vi "Find_Row_Shaft-mm.vi"(0 "Basic Size":dbl, 5 "error in":errorcluster) -> (6 "Row":i32, 8 "error out":errorcluster)   [LabVIEW 2023]
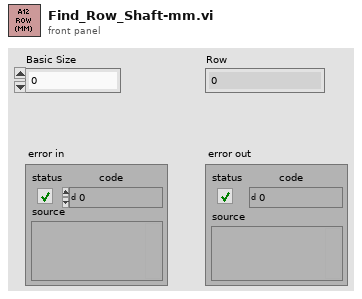
[diagram p1: front panel]
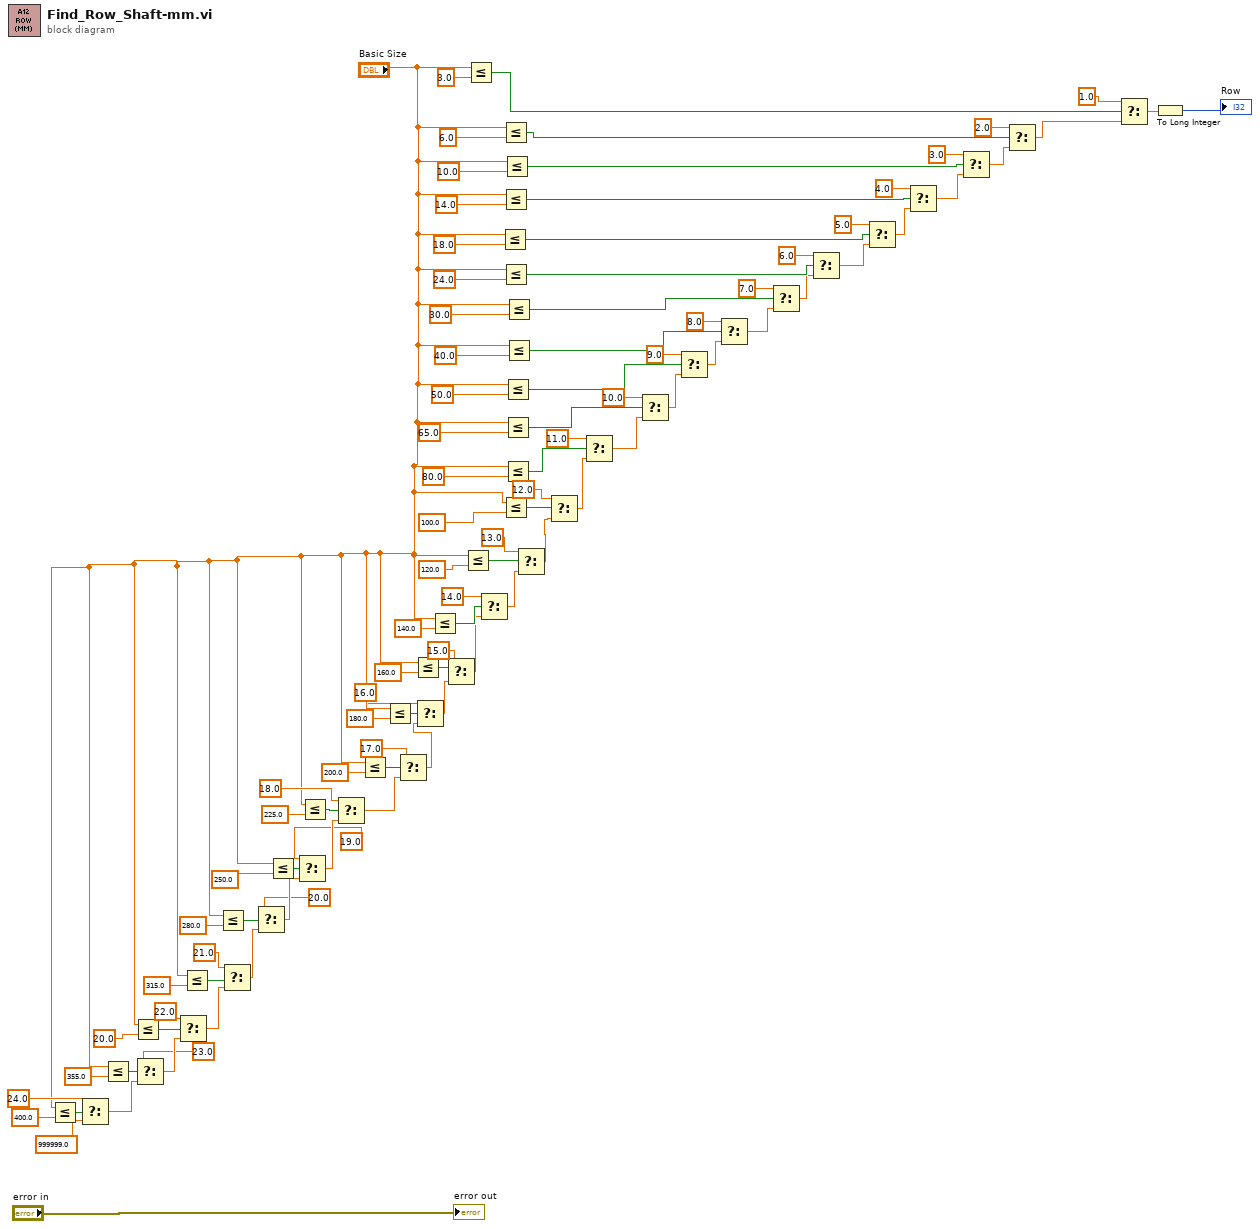
[diagram p0: block diagram]
diagram:
  n1 = Less Or Equal?(x="Basic Size", y=400.0) -> (x <= y?=w8:bool)
  n2 = Select(t=24.0, s=w8, f=999999.0) -> (s? t:f=w10:dbl)
  n3 = Less Or Equal?(x="Basic Size", y=355.0) -> (x <= y?=w13:bool)
  n4 = Less Or Equal?(x="Basic Size", y=20.0 ("t")) -> (x <= y?=w17:bool)
  n5 = Select(t=23.0, s=w13, f=w10) -> (s? t:f=w14:dbl)
  n6 = Select(t=22.0, s=w17, f=w14) -> (s? t:f=w18:dbl)
  n7 = Less Or Equal?(x="Basic Size", y=315.0) -> (x <= y?=w21:bool)
  n8 = Less Or Equal?(x="Basic Size", y=280.0) -> (x <= y?=w25:bool)
  n9 = Select(t=21.0, s=w21, f=w18) -> (s? t:f=w22:dbl)
  n10 = Select(t=20.0, s=w25, f=w22) -> (s? t:f=w26:dbl)
  n11 = Less Or Equal?(x="Basic Size", y=250.0) -> (x <= y?=w29:bool)
  n12 = Select(t=19.0, s=w29, f=w26) -> (s? t:f=w30:dbl)
  n13 = Less Or Equal?(x="Basic Size", y=225.0) -> (x <= y?=w33:bool)
  n14 = Select(t=18.0, s=w33, f=w30) -> (s? t:f=w34:dbl)
  n15 = Less Or Equal?(x="Basic Size", y=200.0) -> (x <= y?=w36:bool)
  n16 = Less Or Equal?(x="Basic Size", y=180.0) -> (x <= y?=w39:bool)
  n17 = Select(t=17.0, s=w36, f=w34) -> (s? t:f=w37:dbl)
  n18 = Less Or Equal?(x="Basic Size", y=160.0) -> (x <= y?=w43:bool)
  n19 = Select(t=16.0, s=w39, f=w37) -> (s? t:f=w40:dbl)
  n20 = Less Or Equal?(x="Basic Size", y=140.0) -> (x <= y?=w46:bool)
  n21 = Select(t=15.0, s=w43, f=w40) -> (s? t:f=w44:dbl)
  n22 = Less Or Equal?(x="Basic Size", y=120.0) -> (x <= y?=w52:bool)
  n23 = Less Or Equal?(x="Basic Size", y=3.0) -> (x <= y?=w99:bool)
  n24 = Select(t=14.0, s=w46, f=w44) -> (s? t:f=w48:dbl)
  n25 = Less Or Equal?(x="Basic Size", y=18.0) -> (x <= y?=w83:bool)
  n26 = Less Or Equal?(x="Basic Size", y=6.0) -> (x <= y?=w95:bool)
  n27 = Less Or Equal?(x="Basic Size", y=14.0) -> (x <= y?=w87:bool)
  n28 = Less Or Equal?(x="Basic Size", y=24.0) -> (x <= y?=w79:bool)
  n29 = Less Or Equal?(x="Basic Size", y=100.0 ("x")) -> (x <= y?=w57:bool)
  n30 = Less Or Equal?(x="Basic Size", y=10.0) -> (x <= y?=w92:bool)
  n31 = Less Or Equal?(x="Basic Size", y=50.0) -> (x <= y?=w67:bool)
  n32 = Less Or Equal?(x="Basic Size", y=65.0) -> (x <= y?=w63:bool)
  n33 = Less Or Equal?(x="Basic Size", y=80.0) -> (x <= y?=w59:bool)
  n34 = Less Or Equal?(x="Basic Size", y=30.0) -> (x <= y?=w75:bool)
  n35 = Less Or Equal?(x="Basic Size", y=40.0) -> (x <= y?=w71:bool)
  n36 = Select(t=13.0, s=w52, f=w48) -> (s? t:f=w51:dbl)
  n37 = Select(t=12.0, s=w57, f=w51) -> (s? t:f=w56:dbl)
  n38 = Select(t=11.0, s=w59, f=w56) -> (s? t:f=w61:dbl)
  n39 = Select(t=10.0, s=w63, f=w61) -> (s? t:f=w66:dbl)
  n40 = Select(t=9.0, s=w67, f=w66) -> (s? t:f=w69:dbl)
  n41 = Select(t=8.0, s=w71, f=w69) -> (s? t:f=w73:dbl)
  n42 = Select(t=7.0, s=w75, f=w73) -> (s? t:f=w77:dbl)
  n43 = Select(t=6.0, s=w79, f=w77) -> (s? t:f=w81:dbl)
  n44 = Select(t=5.0, s=w83, f=w81) -> (s? t:f=w85:dbl)
  n45 = Select(t=4.0, s=w87, f=w85) -> (s? t:f=w89:dbl)
  n46 = Select(t=3.0, s=w92, f=w89) -> (s? t:f=w93:dbl)
  n47 = Select(t=2.0, s=w95, f=w93) -> (s? t:f=w96:dbl)
  n48 = Select(t=1.0, s=w99, f=w96) -> (s? t:f=w53:dbl)
  n49 = To Long Integer(number=w53) -> (32bit integer=→"Row":i32)
  "error out" <- "error in"
